vi "Sleep.vi"(8 "error in":errorcluster, 11 "milliseconds to wait":u32=1000) -> (0 "error out":errorcluster)   [LabVIEW 2021]
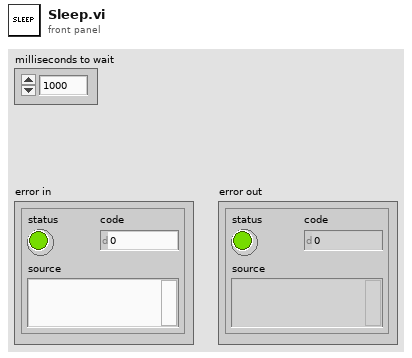
[diagram p1: front panel]
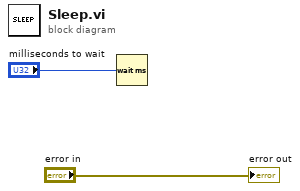
[diagram p0: block diagram]
diagram:
  n1 = Wait (ms)(milliseconds to wait="milliseconds to wait") -> ()  [unwired: 1 out]
  "error out" <- "error in"
